vi "CurrentInputStart.vi"(0 "Device Info":T1={"Serial Number"=-1, "Channel"=0, "Port"=0}, 1 "Data Interval":i32=-1, 2 "Change Trigger":dbl, 11 "error in (no error)":errorcluster, 12 "Connection":u16(ring) items=["No Preference", "Remote", "Local"], 13 "Timeout (mSec)":i32=5000) -> (4 "Phidget ID":u64, 6 "Serial Number Return":i32, 10 "Attached?":bool, 15 "error out":errorcluster)   [LabVIEW 2020, in "Phidget Current Input.lvlib"]
doc: "${CurrentInput:StartHeader}"
uses:
  <instrlib>/Phidgets/Phidget Current Input/Phidget Current Input.lvlib
  <instrlib>/Phidgets/Phidget Common/Phidget Common.lvlib
panel:
  in  "Power Supply":i32(ring)=2 items=["POWER_SUPPLY_OFF"=1, "POWER_SUPPLY_12V"=2, "POWER_SUPPLY_24V"=3]
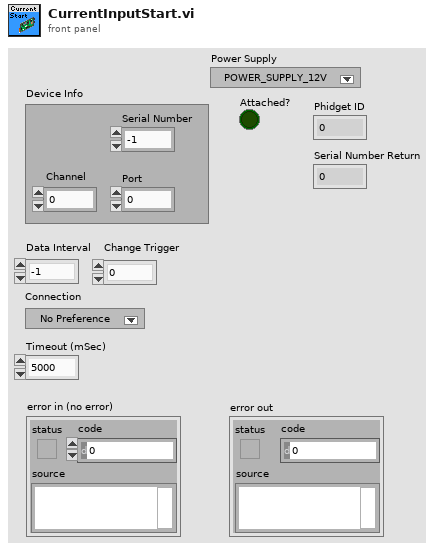
[diagram p1: front panel]
types:
  T1 = cluster{"Serial Number":i32, "Channel":i32, "Port":i32}
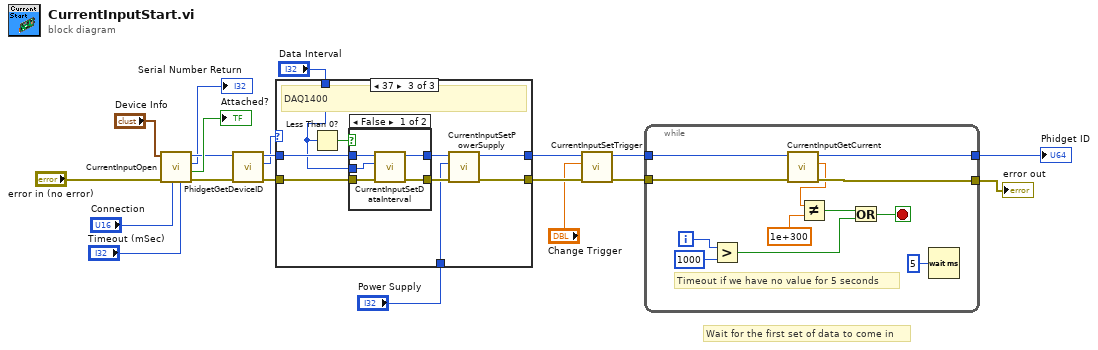
[diagram p0: block diagram]
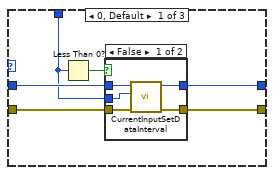
[diagram p2: hidden frame]
diagram:
  # "Wait for the first set of data to come in"
  n1 = call <instrlib>:"CurrentInputOpen.vi"("Timeout (mSec)"="Timeout (mSec)", "Connection"="Connection", "error in"="error in (no error)", "Device Info"="Device Info") -> ("error out"=w17:errorcluster, "Attached?"=→"Attached?":bool, "Serial Number Return"=→"Serial Number Return":i32, "Phidget ID"=w16:u64)  [unwired: 4 in]
  n2 = call <instrlib>:"PhidgetGetDeviceID.vi"("error in (no error)"=w17, "Device In"=w16) -> ("error out"=w14:errorcluster, "Devie IDs"=w13:u32, "Device Out"=w15:u64)  [unwired: 6 in]
  n3 = case shown="37" w13 {
    tunnel: w14 -> [w24 w35 w44]
    tunnel: [w21 w35 w37] -> w7
    tunnel: w15 -> [w26 w34 w43]
    tunnel: [w22 w34 w38] -> w8
    tunnel: "Data Interval" -> [w25 _ w42]
    tunnel: "Power Supply" -> [_ _ w36]
    frame 0, Default {
      n4 = Less Than 0?(x=w25) -> (x < 0?=w23:bool)
      n5 = case shown="False" w23 {
        tunnel: w26 -> [w29 w33]
        tunnel: w24 -> [w31 w32]
        tunnel: w25 -> [w30 _]
        tunnel: [w28 w33] -> w22
        tunnel: [w27 w32] -> w21
        frame False {
          n6 = call <instrlib>:"CurrentInputSetDataInterval.vi"("error in (no error)"=w31, "Interval"=w30, "Device In"=w29) -> ("error out"=w27:errorcluster, "Device Out"=w28:u64)  [unwired: 6 in]
        }
        frame True {
        }
      }
    }
    frame 38, 40..43 {
      # "Do not set\ndata interval on\ndevices that\ndon't support it"
      # "1061, 1063, 1064, 1065, 1066"
    }
    frame 55 {
      # "DAQ1400"
      n7 = Less Than 0?(x=w42) -> (x < 0?=w41:bool)
      n8 = case shown="False" w41 {
        tunnel: w43 -> [w47 w51]
        tunnel: w44 -> [w49 w50]
        tunnel: w42 -> [w48 _]
        tunnel: [w46 w51] -> w39
        tunnel: [w45 w50] -> w40
        frame False {
          n9 = call <instrlib>:"CurrentInputSetDataInterval.vi"("error in (no error)"=w49, "Interval"=w48, "Device In"=w47) -> ("error out"=w45:errorcluster, "Device Out"=w46:u64)  [unwired: 6 in]
        }
        frame True {
        }
      }
      n10 = call <instrlib>:"CurrentInputSetPowerSupply.vi"("error in (no error)"=w40, "Power Supply"=w36, "Device In"=w39) -> ("error out"=w37:errorcluster, "Device Out"=w38:u64)  [unwired: 6 in]
    }
  }
  n11 = call <instrlib>:"CurrentInputSetTrigger.vi"("error in (no error)"=w7, "Trigger"="Change Trigger", "Device In"=w8) -> ("error out"=w9:errorcluster, "Device Out"=w10:u64)  [unwired: 6 in]
  n12 = while {
    tunnel: w10 -> [w61]
    tunnel: w9 -> [w60]
    tunnel: [w58] -> w12
    tunnel: [w59] -> w19
    i -> [w56]
    stop <- w53 stop-if-true
    # "Timeout if we have no value for 5 seconds"
    n13 = Greater?(x=w56, y=1000) -> (0:w54:bool)
    n14 = call <instrlib>:"CurrentInputGetCurrent.vi"("error in (no error)"=w60, "Device In"=w61) -> ("error out"=w59:errorcluster, "Current"=w52:dbl, "Device Out"=w58:u64)  [unwired: 6 in]
    n15 = Not Equal?(x=w52, y=1e+300) -> (x != y?=w55:bool)
    n16 = Or(x=w55, y=w54) -> (x .or. y?=w53:bool)
    n17 = Wait (ms)(milliseconds to wait=u32 5) -> ()  [unwired: 1 out]
  }
  "error out" <- w19
  "Phidget ID" <- w12
